vi "Dispense FN - ON (SubVI).vi"(0 "Signals IN":T3, 1 "Values IN":T2 {"Drain Time (s)" format="%.2f"; "Drain Rate (g/sec)" format="%.2f"}, 2 "Settings":T1={"ON Settings"={"Enable Dynamic Setpoint?"=TRUE, "Enable Dynamic Dispense Time?"=TRUE, "Enable Drain Rate Functions"=TRUE, "Dispense Sample Time (s)"=0.5, "Dispense Slope Ave"=0, "ON Timeout (sec)"=600.0, "1st Setpoint (% of Target)"=0.0, "2nd Setpoint (% of Target)"=0.0, "3rd Setpoint (% of Target)"=0.0, "Measure Dispense Delay (sec)"=0.0, "Settle Slope Sample Time (s)"=0.0}, "OFF Settings"={"Drain Sample Time (s)"=0.5, "Drain Rate Ave Size"=5, "Drain Rate Limits (± g/sec)"=10.0, "Level Slope Range (± g/sec)"=0.25, "OFF Timeout (sec)"=0.0, "Near SP Slope Level (± g/sec)"=0.01, "Near Setpoint Threshold (%)"=95.0}, "Overshoot Settings"={"Time Limit (s)"=60.0, "Container MAX (g)"=1500.0, "Max FILL Slope (+/- g/sec)"=10.0, "% Overshot to Enable (>)"=0.25}, "FILL Timeout (s)"=300.0, "Full Settle Time (s)"=20.0, "Pre-Hydrate \nSpray Time (s)"=10.0, "Pre-Hydrate \nWait Time (s)"=30.0}, 3 "Main Concentration Setpoint (%)":dbl, 4 "Measured Mass (g)":dbl, 5 "State Change?":bool, 7 "Main Case Change?":bool) -> (14 "Signals OUT":T3, 15 "Values OUT":T2 {"Drain Time (s)" format="%.2f"; "Drain Rate (g/sec)" format="%.2f"}, 17 "Spray Count":i32, 19 "OFF Signal":bool)   [LabVIEW 2009]
uses:
  <vilib>/ptbypt/NI_PtbyPt.lvlib
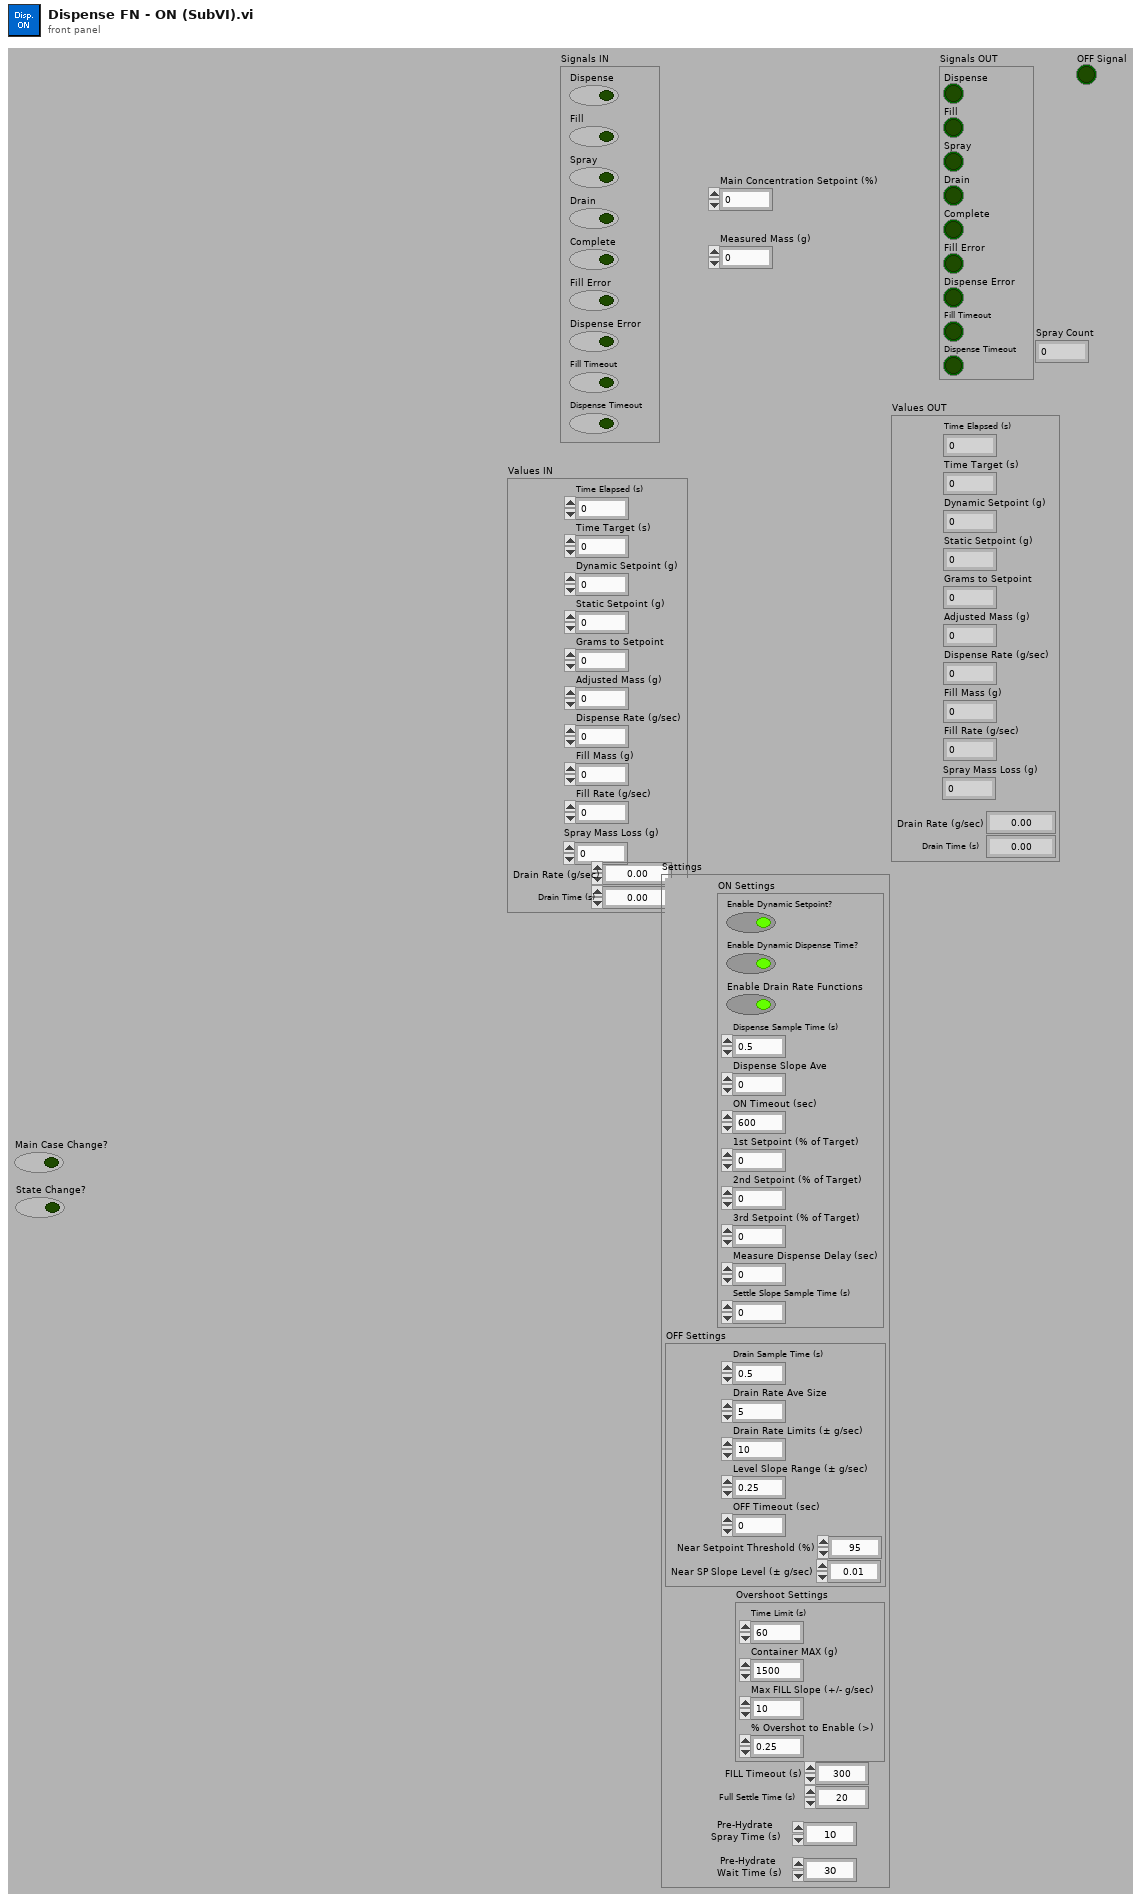
[diagram p1: front panel]
types:
  T1 = cluster{"ON Settings":cluster{"Enable Dynamic Setpoint?":bool, "Enable Dynamic Dispense Time?":bool, "Enable Drain Rate Functions":bool, "Dispense Sample Time (s)":dbl, "Dispense Slope Ave":i32, "ON Timeout (sec)":dbl, "1st Setpoint (% of Target)":dbl, "2nd Setpoint (% of Target)":dbl, "3rd Setpoint (% of Target)":dbl, "Measure Dispense Delay (sec)":dbl, "Settle Slope Sample Time (s)":dbl}, "OFF Settings":cluster{"Drain Sample Time (s)":dbl, "Drain Rate Ave Size":i32, "Drain Rate Limits (± g/sec)":dbl, "Level Slope Range (± g/sec)":dbl, "OFF Timeout (sec)":dbl, "Near SP Slope Level (± g/sec)":dbl, "Near Setpoint Threshold (%)":dbl}, "Overshoot Settings":cluster{"Time Limit (s)":dbl, "Container MAX (g)":dbl, "Max FILL Slope (+/- g/sec)":dbl, "% Overshot to Enable (>)":dbl}, "FILL Timeout (s)":dbl, "Full Settle Time (s)":dbl, "Pre-Hydrate \nSpray Time (s)":dbl, "Pre-Hydrate \nWait Time (s)":dbl}
  T2 = cluster{"Time Elapsed (s)":dbl, "Time Target (s)":dbl, "Dynamic Setpoint (g)":dbl, "Static Setpoint (g)":dbl, "Grams to Setpoint":dbl, "Adjusted Mass (g)":dbl, "Dispense Rate (g/sec)":dbl, "Fill Mass (g)":dbl, "Fill Rate (g/sec)":dbl, "Spray Mass Loss (g)":dbl, "Drain Rate (g/sec)":dbl, "Drain Time (s)":dbl}
  T3 = cluster{"Dispense":bool, "Fill":bool, "Spray":bool, "Drain":bool, "Complete":bool, "Fill Error":bool, "Dispense Error":bool, "Fill Timeout":bool, "Dispense Timeout":bool}
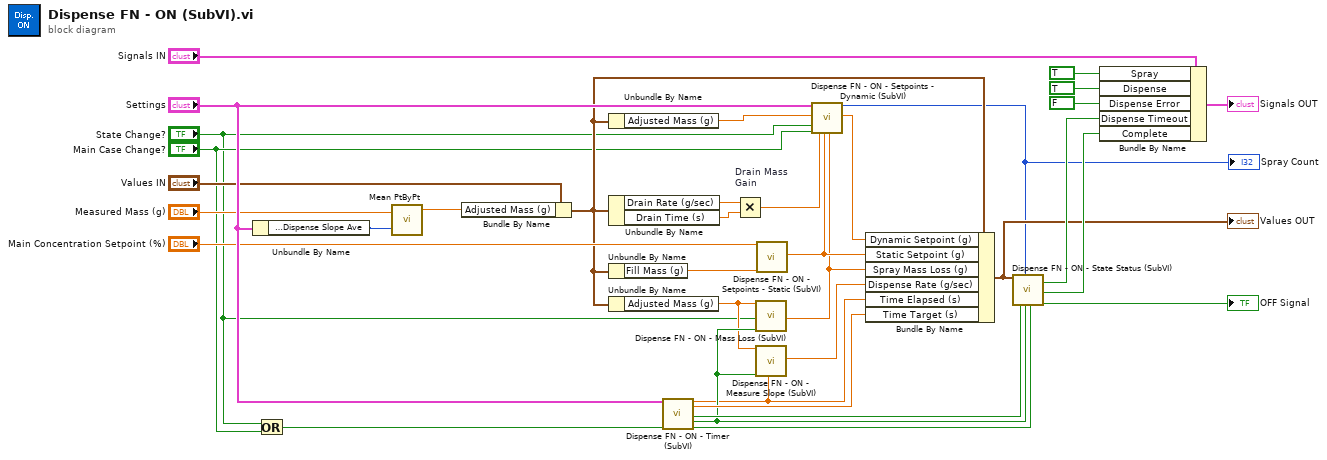
[diagram p0: block diagram]
diagram:
  n1 = Unbundle By Name("Settings") -> ("ON Settings.Dispense Slope Ave"=w18:i32)
  n2 = Or(x="State Change?", y="Main Case Change?") -> (x .or. y?=w3:bool)
  n3 = call <vilib>:"Mean PtByPt.vi"("x"="Measured Mass (g)", "sample length"=w18) -> ("mean"=w21:dbl)  [unwired: 1 in, 2 out]
  n4 = Bundle By Name(cluster="Values IN", "Adjusted Mass (g)"=w21) -> (w6:T2)
  n5 = Unbundle By Name(w6) -> ("Adjusted Mass (g)"=w20:dbl)
  n6 = Unbundle By Name(w6) -> ("Drain Rate (g/sec)"=w26:dbl, "Drain Time (s)"=w25:dbl)
  n7 = Unbundle By Name(w6) -> ("Fill Mass (g)"=w27:dbl)
  n8 = Unbundle By Name(w6) -> ("Adjusted Mass (g)"=w8:dbl)
  n9 = call "Dispense FN - ON - Timer (SubVI).vi"("Settings"="Settings", "Reset"=w3) -> ("Elapsed Time (s)"=w7:dbl, "ON Timeout (s)"=w17:dbl, "Min Spray Complete?"=w12:bool, "Measure Delay Complete?"=w11:bool, "Max Spray Complete?"=w10:bool)  [unwired: 13 in]
  n10 = Multiply "Drain Mass\nGain"(x=w26, y=w25) -> (x*y=w24:dbl)
  n11 = call "Dispense FN - ON - Mass Loss (SubVI).vi"("Measured Mass (g)"=w8, "State Change?"="State Change?", "Measure Delay Complete?"=w11) -> ("Dispense Mass Loss"=w22:dbl)  [unwired: 16 in]
  n12 = call "Dispense FN - ON - Measure Slope (SubVI).vi"("Measured Mass (g)"=w8, "Measure Delay Complete?"=w11, "Elapsed Time (s)"=w7) -> ("Ave. Slope (g/sec)"=w9:dbl)  [unwired: 16 in]
  n13 = call "Dispense FN - ON - Setpoints - Static (SubVI).vi"("Main Concentration Setpoint (%)"="Main Concentration Setpoint (%)", "Fill Mass (g)"=w27) -> ("Static Setpoint (g)"=w23:dbl)  [unwired: 17 in]
  n14 = call "Dispense FN - ON - Setpoints - Dynamic (SubVI).vi"("Settings"="Settings", "Measured Mass (g)"=w20, "State Change?"="State Change?", "Main Case Change?"="Main Case Change?", "Drain Mass Gain (g)"=w24, "Static Setpoint (g)"=w23, "Spray Mass Loss (g)"=w22) -> ("Spray Count"=w1:i32, "Dynamic Setpoint (g)"=w29:dbl)  [unwired: 11 in]
  "Spray Count" <- w1
  n15 = Bundle By Name(cluster=w6, "Dynamic Setpoint (g)"=w29, "Static Setpoint (g)"=w23, "Spray Mass Loss (g)"=w22, "Dispense Rate (g/sec)"=w9, "Time Elapsed (s)"=w7, "Time Target (s)"=w17) -> (w5:T2)
  "Values OUT" <- w5
  n16 = call "Dispense FN - ON - State Status (SubVI).vi"("Values IN"=w5, "Min Spray Complete?"=w12, "Spray Count"=w1, "Measure Delay Complete?"=w11, "Max Spray Complete?"=w10) -> ("Dispense Timeout?"=w16:bool, "Complete"=w15:bool, "OFF Signal"=→"OFF Signal":bool)  [unwired: 8 in, 4 out]
  n17 = Bundle By Name(cluster="Signals IN", "Spray"=TRUE, "Dispense"=TRUE, "Dispense Error"=FALSE, "Dispense Timeout"=w16, "Complete"=w15) -> (→"Signals OUT":T3)
